vi "Write HDI Picked.vi"(8 "error in (no error)":errorcluster, 10 "HDI Picked":bool, 11 "PickerTool Class in":refnum<class "PickerTool Class.lvclass">) -> (0 "error out":errorcluster, 3 "PickerTool Class out":refnum<class "PickerTool Class.lvclass">)   [LabVIEW 2017, in "PickerTool Class.lvclass"]
uses:
  PickerTool Class.lvclass
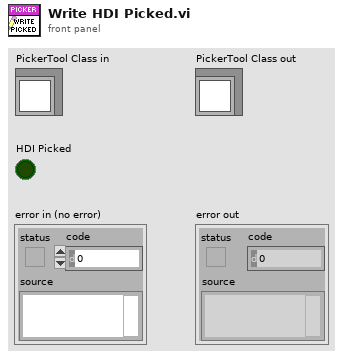
[diagram p1: front panel]
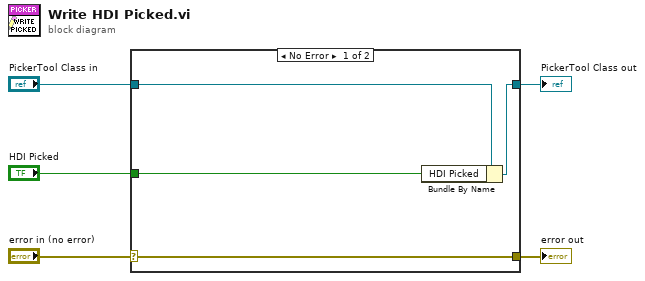
[diagram p0: block diagram]
diagram:
  n1 = case shown="No Error" "error in (no error)" {
    selector: "error in (no error)" -> [w9 w10]
    tunnel: [w9 w10] -> w4
    tunnel: [w7 w11] -> w2
    tunnel: "PickerTool Class in" -> [w8 w11]
    tunnel: "HDI Picked" -> [w6 _]
    frame No Error {
      n2 = Bundle By Name(cluster=w8, "HDI Picked"=w6) -> (w7:refnum<class "PickerTool Class.lvclass">)
    }
    frame Error {
    }
  }
  "error out" <- w4
  "PickerTool Class out" <- w2
